vi "Initialize.vi"(8 "Interior cargo capacity":dbl, 9 "model":string, 10 "make":string, 11 "vehicle in":refnum<class "Vehicle.lvclass">) -> (3 "vehicle out":refnum<class "Vehicle.lvclass">)   [LabVIEW 2020, in "Vehicle.lvclass"]
doc: "This method initializes the data members of the Vehicle class."
uses:
  Vehicle.lvclass
  Vehicle.lvclass/Vehicle.ctl
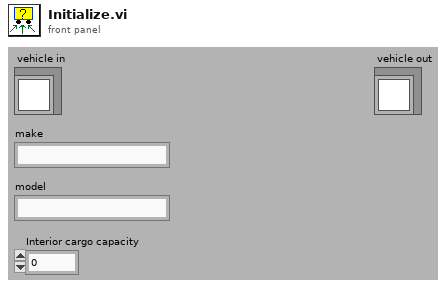
[diagram p1: front panel]
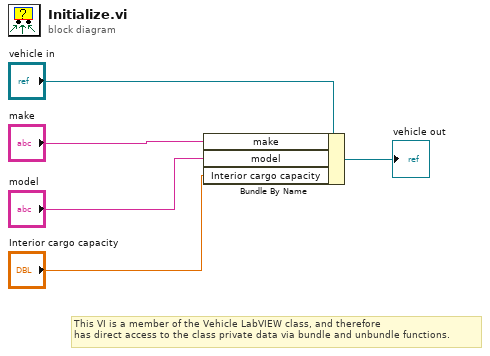
[diagram p0: block diagram]
diagram:
  # "This VI is a member of the Vehicle LabVIEW class, and therefore\nhas direct access to the class private data via bundle and unbundle functions."
  n1 = Bundle By Name(cluster="vehicle in", "make"="make", "model"="model", "Interior cargo capacity"="Interior cargo capacity") -> (→"vehicle out":refnum<class "Vehicle.lvclass">)
